vi "Method Quaking.vi"(8 "error in (no error)":errorcluster, 11 "Quacking Behaviors in":refnum<class "Quacking Behaviors.lvclass">) -> (0 "error out":errorcluster, 3 "Quacking Behaviors out":refnum<class "Quacking Behaviors.lvclass">)   [LabVIEW 2021, in "Quacking Behaviors.lvclass"]
uses:
  Quacking Behaviors.lvclass
  Quacking Behaviors.lvclass/Quacking Behaviors.ctl
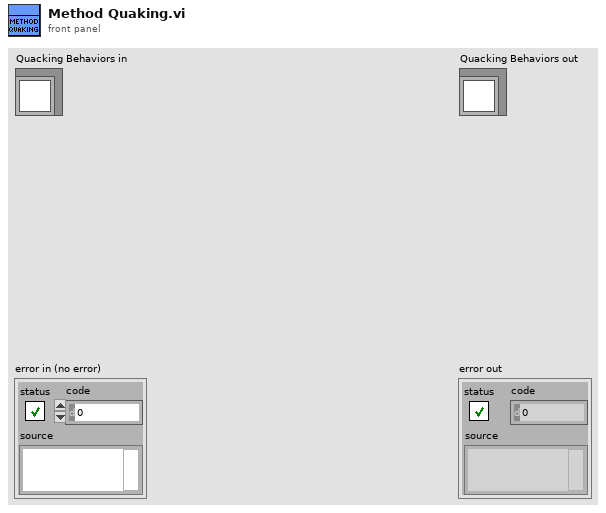
[diagram p1: front panel]
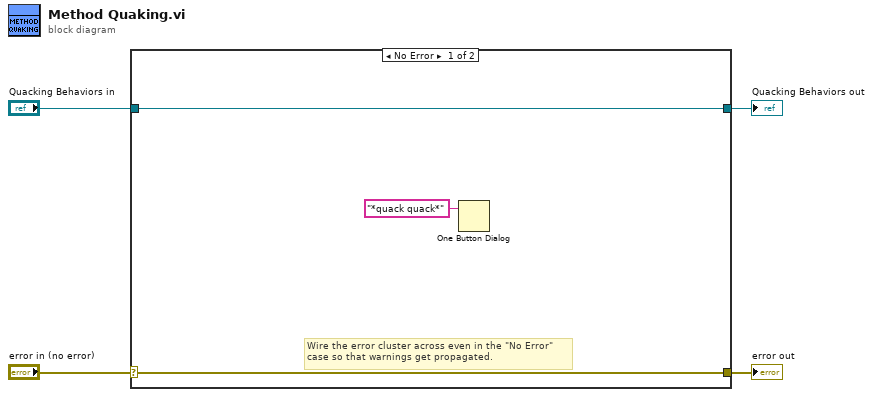
[diagram p0: block diagram]
diagram:
  n1 = case shown="No Error" "error in (no error)" {
    selector: "error in (no error)" -> [w6 w9]
    tunnel: [w6 w9] -> w3
    tunnel: [w7 w8] -> w1
    tunnel: "Quacking Behaviors in" -> [w7 w8]
    frame No Error {
      # "Wire the error cluster across even in the \"No Error\"\ncase so that warnings get propagated."
      n2 = One Button Dialog(message="*quack quack*") -> ()  [unwired: 1 in, 1 out]
    }
    frame Error {
    }
  }
  "error out" <- w3
  "Quacking Behaviors out" <- w1
